vi "QSM Counting Example.vi"() -> ()   [LabVIEW 2020]
uses:
  States.ctl
panel:
  in  "Max Value":dbl=50.0
  in  "stop":bool
  in  "Start":bool
  out "Waveform Chart":dbl(graph)=4.228293507567721
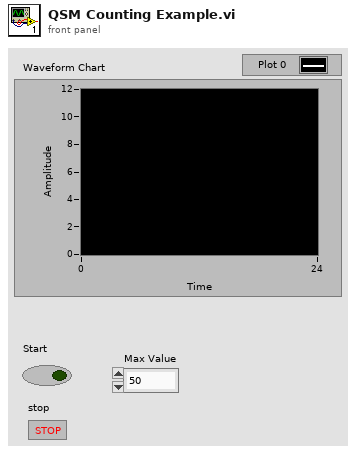
[diagram p1: front panel]
types:
  T1 = typedef "States.ctl" = enum16{"Stop", "Initialize", "Add to Plot", "Add More Data", "Idle 1", "Idle 2"}
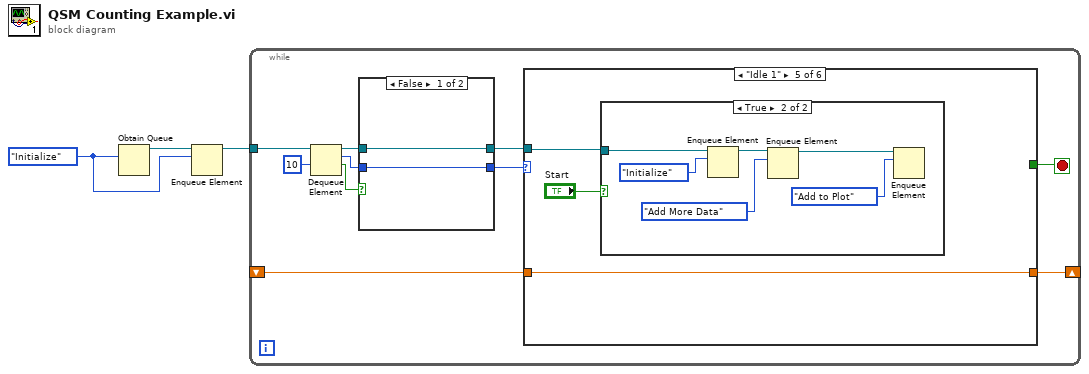
[diagram p0: block diagram]
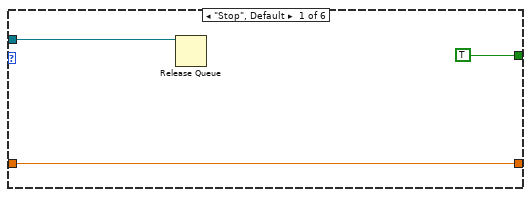
[diagram p2: hidden frame]
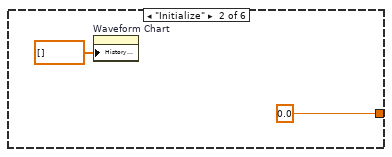
[diagram p3: hidden frame]
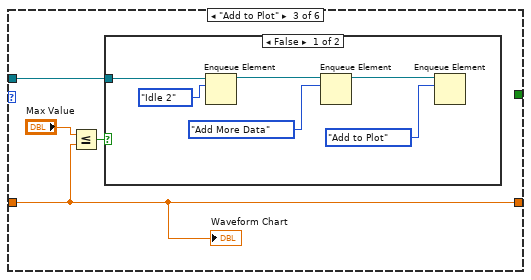
[diagram p4: hidden frame]
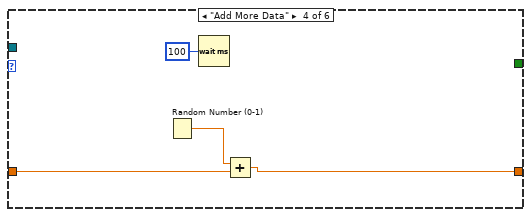
[diagram p6: hidden frame]
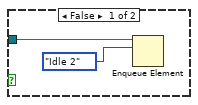
[diagram p7: hidden frame]
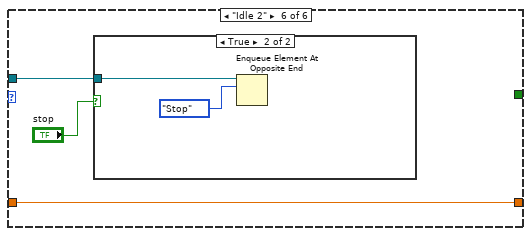
[diagram p8: hidden frame]
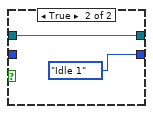
[diagram p10: hidden frame]
diagram:
  w2 = States."Initialize"
  n1 = Obtain Queue(element data type=w2) -> (queue out=w3:refnum<queue>)  [unwired: 4 in, 2 out]
  n2 = Enqueue Element(queue=w3, element=w2) -> (queue out=w1:refnum<queue>)  [unwired: 2 in, 2 out]
  n3 = while {
    tunnel: w1 -> [w13]
    shift-right: [w6] -> _
    shift-left: _ -> [w5]
    stop <- w4 stop-if-true
    n4 = Dequeue Element(queue=w13, timeout in ms (-1)=10) -> (queue out=w10:refnum<queue>, element=w8:T1, timed out?=w11:bool)  [unwired: 1 in, 1 out]
    n5 = case shown="False" w11 {
      tunnel: w10 -> [w49 w52]
      tunnel: [w49 w52] -> w7
      tunnel: [w50 States."Idle 1"] -> w9
      tunnel: w8 -> [w50 _]
      frame False {
      }
      frame True {
      }
    }
    n6 = case shown="\"Idle 1\"" w9 {
      tunnel: w7 -> [w15 _ w20 _ w34 w45]
      tunnel: [w14 0.0 w19 w30 w33 w44] -> w6
      tunnel: w5 -> [w14 _ w19 w31 w33 w44]
      tunnel: [TRUE _ _ _ _ _] -> w4
      frame "Stop", Default {
        n7 = Release Queue(queue=w15) -> ()  [unwired: 2 in, 3 out]
      }
      frame "Initialize" {
        n8 = property on="Waveform Chart" class="WFChart (strict)"("History Data"=dbl[] []) -> ()  [unwired: 2 in, 2 out]
      }
      frame "Add to Plot" {
        n9 = Less Or Equal?(x="Max Value", y=w19) -> (x <= y?=w21:bool)
        n10 = case shown="False" w21 {
          tunnel: w20 -> [w28 _]
          frame False {
            n11 = Enqueue Element(queue=w28, element=States."Idle 2") -> (queue out=w26:refnum<queue>)  [unwired: 2 in, 2 out]
            n12 = Enqueue Element(queue=w26, element=States."Add More Data") -> (queue out=w24:refnum<queue>)  [unwired: 2 in, 2 out]
            n13 = Enqueue Element(queue=w24, element=States."Add to Plot") -> ()  [unwired: 2 in, 3 out]
          }
          frame True {
          }
        }
        "Waveform Chart" <- w19
      }
      frame "Add More Data" {
        n14 = Random Number (0-1)() -> (number: 0 to 1=w32:dbl)
        n15 = Wait (ms)(milliseconds to wait=u32 100) -> ()  [unwired: 1 out]
        n16 = Add(x=w32, y=w31) -> (x+y=w30:dbl)
      }
      frame "Idle 1" {
        n17 = case shown="True" "Start" {
          tunnel: w34 -> [w37 w42]
          frame False {
            n18 = Enqueue Element(queue=w37, element=States."Idle 2") -> ()  [unwired: 2 in, 3 out]
          }
          frame True {
            n19 = Enqueue Element(queue=w42, element=States."Initialize") -> (queue out=w41:refnum<queue>)  [unwired: 2 in, 2 out]
            n20 = Enqueue Element(queue=w41, element=States."Add More Data") -> (queue out=w39:refnum<queue>)  [unwired: 2 in, 2 out]
            n21 = Enqueue Element(queue=w39, element=States."Add to Plot") -> ()  [unwired: 2 in, 3 out]
          }
        }
      }
      frame "Idle 2" {
        n22 = case shown="True" "stop" {
          tunnel: w45 -> [_ w48]
          frame False {
          }
          frame True {
            n23 = Enqueue Element At Opposite End(queue=w48, element=States."Stop") -> ()  [unwired: 2 in, 3 out]
          }
        }
      }
    }
  }
